vi "uber encoder2.vi"(5 "EncoderDevRef":T1={"DevStatus"={"status"=FALSE, "code"=0, "source"=""}, "EncoderIndex"=enum."Invalid", "CounterIndex"=enum."Ctr 1", "DistancePerCount"=2.0, "Decoding Type"=enum."4x"}) -> (0 "rate":dbl, 1 "Distance":dbl, 2 "EncoderDevRef out":T1={"DevStatus"={"status"=FALSE, "code"=0, "source"=""}, "EncoderIndex"=enum."Invalid", "CounterIndex"=enum."Ctr 1", "DistancePerCount"=2.0, "Decoding Type"=enum."4x"})   [LabVIEW 2011]
uses:
  <vilib>/Rock Robotics/WPI/Encoder/WPI_EncoderDevRef.ctl
  <vilib>/Rock Robotics/SystemInterfaces/Encoder/FPGA_EncoderIdx.ctl
  <vilib>/Rock Robotics/SystemInterfaces/Counter/FPGA_CounterCtrSystemIndex.ctl
  <vilib>/Rock Robotics/WPI/Encoder/WPI_EncoderType.ctl
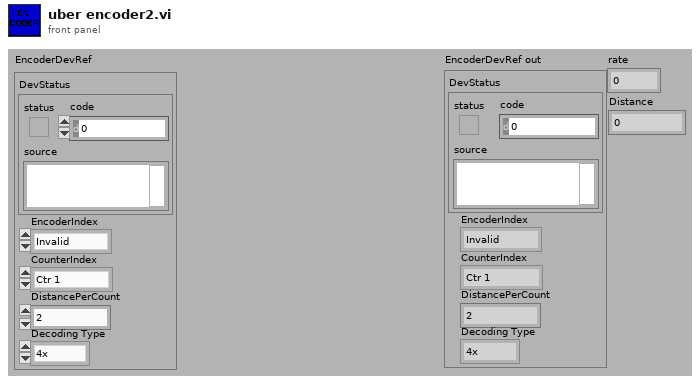
[diagram p1: front panel]
types:
  T1 = typedef "WPI_EncoderDevRef.ctl" = cluster{"DevStatus":errorcluster, "EncoderIndex":T2, "CounterIndex":T3, "DistancePerCount":dbl, "Decoding Type":T4}
  T2 = typedef "FPGA_EncoderIdx.ctl" = enum8{"Enc 0", "Enc 1", "Enc 2", "Enc 3", "Invalid"}
  T3 = typedef "FPGA_CounterCtrSystemIndex.ctl" = enum8{"Ctr 0", "Ctr 1", "Ctr 2", "Ctr 3", "Ctr 4", "Ctr 5", "Ctr 6", "Ctr 7", "Invalid"}
  T4 = typedef "WPI_EncoderType.ctl" = enum16{"1x", "2x", "4x"}
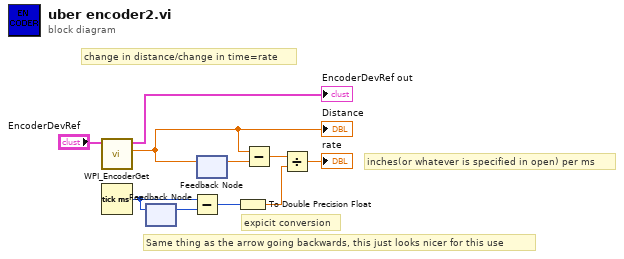
[diagram p0: block diagram]
diagram:
  # "change in distance/change in time=rate"
  # "expicit conversion"
  # "Same thing as the arrow going backwards, this just looks nicer for this use"
  # "inches(or whatever is specified in open) per ms"
  n1 = call <vilib>:"WPI_EncoderGet.vi"("EncoderDevRef"="EncoderDevRef") -> ("Distance"=w5:dbl, "EncoderDevRef"=→"EncoderDevRef out":T1)  [unwired: 1 in, 8 out]
  "Distance" <- w5
  n2 = Tick Count (ms)() -> (millisecond timer value=w10:u32)
  n3 = feedback-in #1(w10) -> ()
  n4 = feedback #1() -> (w9:u32)  [unwired: 1 out]
  n5 = Subtract(x=w10, y=w9) -> (x-y=w2:u32)
  n6 = feedback-in #2(w5) -> ()
  n7 = feedback #2() -> (w4:dbl)  [unwired: 1 out]
  n8 = To Double Precision Float(number=w2) -> (double precision float=w1:dbl)
  n9 = Subtract(x=w5, y=w4) -> (x-y=w6:dbl)
  n10 = Divide(x=w6, y=w1) -> (x/y=→"rate":dbl)
